vi "Get LabVIEW Version.vi"(11 "Project Version String":string) -> (1 "Version (numeric) out":i32, 3 "Version (string) out":string)   [LabVIEW 2015, in "LV Project Version Check.lvlib"]
uses:
  LV Project Version Check.lvlib
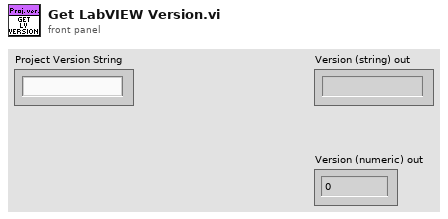
[diagram p1: front panel]
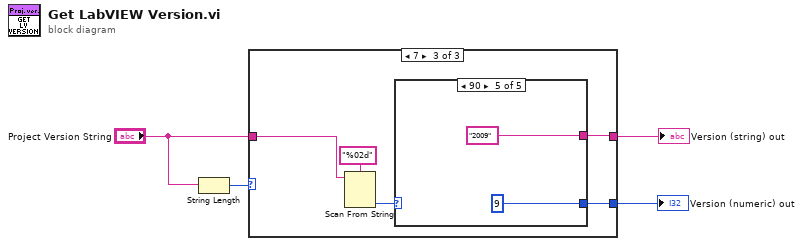
[diagram p0: block diagram]
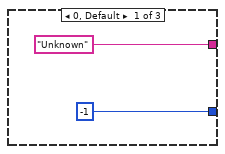
[diagram p2: hidden frame]
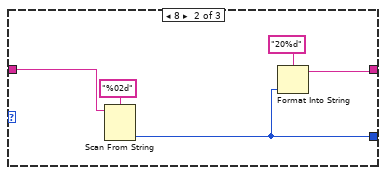
[diagram p3: hidden frame]
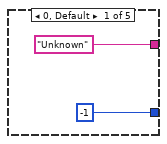
[diagram p4: hidden frame]
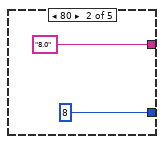
[diagram p5: hidden frame]
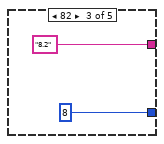
[diagram p6: hidden frame]
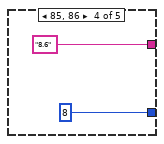
[diagram p7: hidden frame]
diagram:
  n1 = String Length(string="Project Version String") -> (length=w4:i32)
  n2 = case shown="7" w4 {
    tunnel: "Project Version String" -> [_ w10 w15]
    tunnel: ["Unknown" ("Project Version String") w9 w13] -> w2
    tunnel: [-1 w8 w12] -> w1
    frame 0, Default {
    }
    frame 8 {
      n3 = Scan From String(format string="%02d", input string=w10) -> (output 1=w8:i32)  [unwired: 3 in, 3 out]
      n4 = Format Into String(format string="20%d", w8) -> (resulting string=w9:string)  [unwired: 2 in, 1 out]
    }
    frame 7 {
      n5 = Scan From String(format string="%02d", input string=w15) -> (output 1=w14:i32)  [unwired: 3 in, 3 out]
      n6 = case shown="90" w14 {
        tunnel: ["Unknown" "8.0" "8.2" "8.6" "2009"] -> w13
        tunnel: [-1 8 8 8 9] -> w12
        frame 0, Default {
        }
        frame 80 {
        }
        frame 82 {
        }
        frame 85, 86 {
        }
        frame 90 {
        }
      }
    }
  }
  "Version (string) out" <- w2
  "Version (numeric) out" <- w1
